vi "test - copy state with Skip option.vi"(8 "error in (no error)":errorcluster, 11 "TestCase in":refnum<class "testcase-csmhelper.lvclass">) -> (0 "error out":errorcluster, 3 "TestCase out":refnum<class "testcase-csmhelper.lvclass">)   [LabVIEW 2017, in "testcase-csmhelper.lvclass"]
uses:
  testcase-csmhelper.lvclass
  <vilib>/addons/_JKI Toolkits/VI Tester/TestCase.llb/TestCase.lvclass
  src/user.lib/_NEVSTOP/Communicable State Machine(CSM)/Communicable State Machine.lvlib
  C:/Program Files (x86)/National Instruments/LabVIEW 2017/vi.lib/addons/_JKI Toolkits/VI Tester/TestCase.llb/TestCase.lvclass
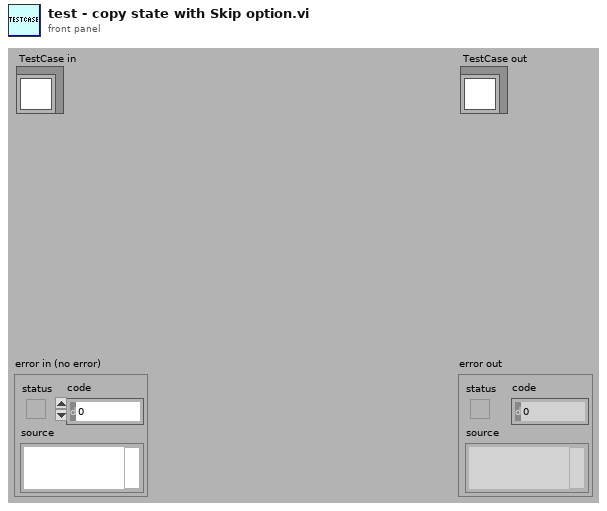
[diagram p1: front panel]
types:
  T1 = enum32{"Bad", "Idle", "Run top level", "Running"}
  T2 = cluster{"state":string, "error out":errorcluster, "Execution:State":enum32{"Bad", "Idle", "Run top level", "Running"}}[]
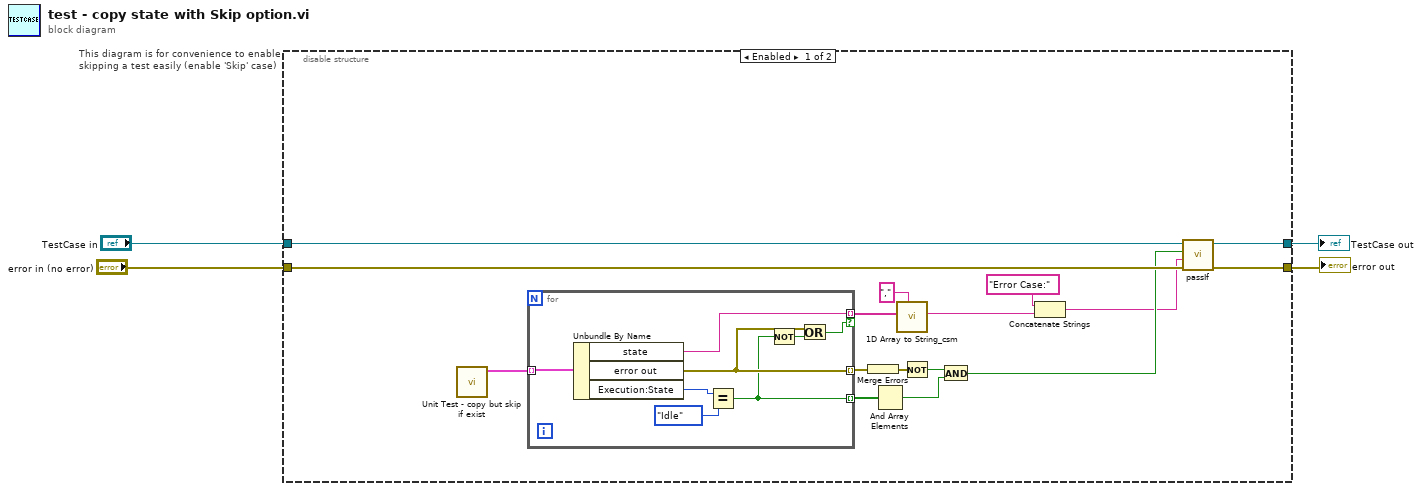
[diagram p0: block diagram]
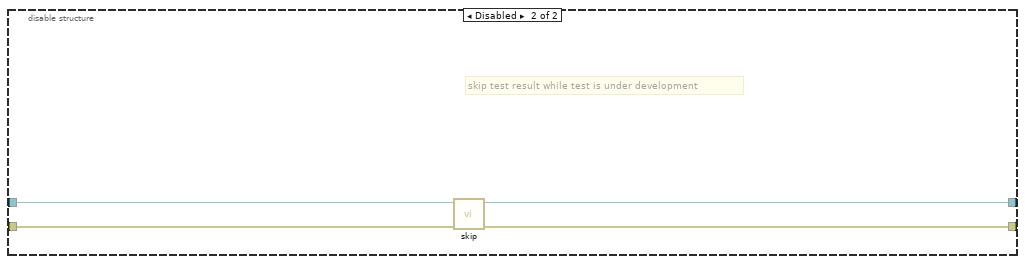
[diagram p2: hidden frame]
diagram:
  n1 = disable-structure "This diagram is for convenience to enable skipping a test easily (enable 'Skip' case)" shown="Enabled" {
    disable-tunnel: "TestCase in" -> [w14 w32]
    disable-tunnel: [w13 w30] -> w1
    disable-tunnel: [w11 w31] -> w3
    disable-tunnel: "error in (no error)" -> [w12 w29]
    frame Enabled {
      n2 = call "Unit Test - copy but skip if exist.vi"() -> ("Array"=w20:T2)  [unwired: 11 in]
      n3 = for {
        tunnel: w20 -> [w28] mode=indexing
        tunnel: [w24] -> w18 mode=indexing
        tunnel: [w22] -> w19 mode=indexing
        tunnel: [w25] -> w9 mode=indexing if=w23
        n4 = Unbundle By Name(w28) -> ("state"=w25:string, "error out"=w24:errorcluster, "Execution:State"=w27:T1)
        n5 = Equal?(x=w27, y=T1."Idle") -> (x = y?=w22:bool)
        n6 = Not(x=w22) -> (.not. x?=w21:bool)
        n7 = Or(x=w24, y=w21) -> (x .or. y?=w23:bool)
      }
      n8 = Merge Errors(w18) -> (w17:errorcluster)
      n9 = And Array Elements(Boolean array=w19) -> (logical AND=w15:bool)
      n10 = call "1D Array to String_csm.vi"("delimiter (Tab)"=",", "Array of Strings"=w9) -> ("delimited string"=w8:string)  [unwired: 9 in]
      n11 = Not(x=w17) -> (.not. x?=w16:bool)
      n12 = And(x=w16, y=w15) -> (x .and. y?=w10:bool)
      n13 = Concatenate Strings("Error Case:" ("string"), w8) -> (w6:string)
      n14 = call-dynamic "passIf.vi"("error in (no error)"=w12, "message (\"\")"=w6, "pass"=w10, "TestCase in"=w14) -> ("error out"=w11:errorcluster, "TestCase out"=w13:refnum<class "testcase-csmhelper.lvclass">)  [unwired: 6 in]
    }
    frame Disabled {
      # "skip test result while test is under development"
      n15 = call <vilib>:"skip.vi"("error in (no error)"=w29, "TestCase in"=w32) -> ("error out"=w31:errorcluster, "TestCase out"=w30:refnum<class "testcase-csmhelper.lvclass">)  [unwired: 8 in]
    }
  }
  "error out" <- w3
  "TestCase out" <- w1
